vi "Cleanup.vi"(8 "error in (no error)":errorcluster, 11 "TCP Server in":refnum<class "TCP Server.lvclass">) -> (0 "error out":errorcluster)   [LabVIEW 2012, in "Stream-TCP.lvlib" / "TCP Server.lvclass"]
uses:
  TCP Server.lvclass
  lv-stream/stream/Endpoint/Endpoint.lvclass
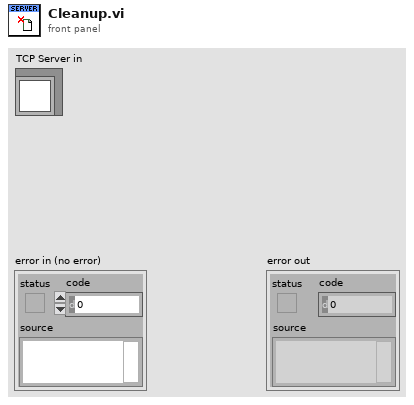
[diagram p1: front panel]
types:
  T1 = typedef "Stream-TCP.lvlib/Listener Notifier.ctl" = refnum<notifier>
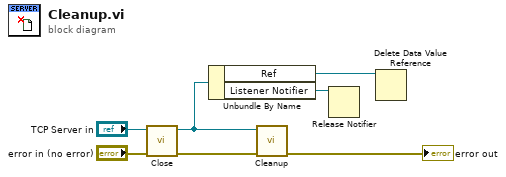
[diagram p0: block diagram]
diagram:
  n1 = call-dynamic "Close.vi"("error in (no error)"="error in (no error)", "TCP Server in"="TCP Server in") -> ("error out"=w4:errorcluster, "TCP Server out"=w3:refnum<class "TCP Server.lvclass">)  [unwired: 8 in]
  n2 = Unbundle By Name(w3) -> ("Ref"=w1:refnum<data-value>, "Listener Notifier"=w2:T1)
  n3 = call-parent "Cleanup.vi"("error in (no error)"=w4, "Endpoint in"=w3) -> ("error out"=→"error out":errorcluster)  [unwired: 9 in]
  n4 = Release Notifier(notifier=w2) -> ()  [unwired: 2 in, 3 out]
  n5 = Delete Data Value Reference(data value reference=w1) -> ()  [unwired: 1 in, 2 out]
